vi "split_averaging_filter_cdb.vi"(4 "Reset":bool, 8 "Parameters":T1={"Order"=0, "Time constant"=0.0, "Detrend mode"=enum."Robust linear", "TD amplitude limit"=inf, "FFT filter"=TRUE, "Notch channels"=[], "LF cutoff"=0, "FD amplitude limit"=0.0}, 9 "Noise":bool, 11 "Error":cdb[](array[numeric])) -> (1 "Model":cdb[](array[numeric]) format="%#_3p", 3 "Prediction":cdb[](array[numeric]) format="%#_4p")   [LabVIEW 2014]
uses:
  averaging_filter_params.ctl
  detrend_mode.ctl
panel:
  # "Prediction for next data block, the same size as our input this time."
  # "The filter tracking error (what we are to try to cancel)."
  # "The time domain model, with length \"Order\".   This is synchronous with the repeat period."
  # "If true, our adaptation should be suppressed on this \"Signal\" block."
  # "This is derived from split_averaging_filter_nu.vi, but has been modified to work with complex input/output data, with inputs that have DC component, and some unused features have also been deleted."
  # "Reset clears state to zeroes.  Filter must then settle to the steady-state output (multiple time constants)."
  # "Model of a repeating signal with known repeat period (order).  Input may be any length; prediction is the same size as input, while the model is of the specified order.  This is like the averaging function on an oscilloscope.  As long as the time constant is much longer than the filter order, only signals that are synchronous with the order pass through into the model."
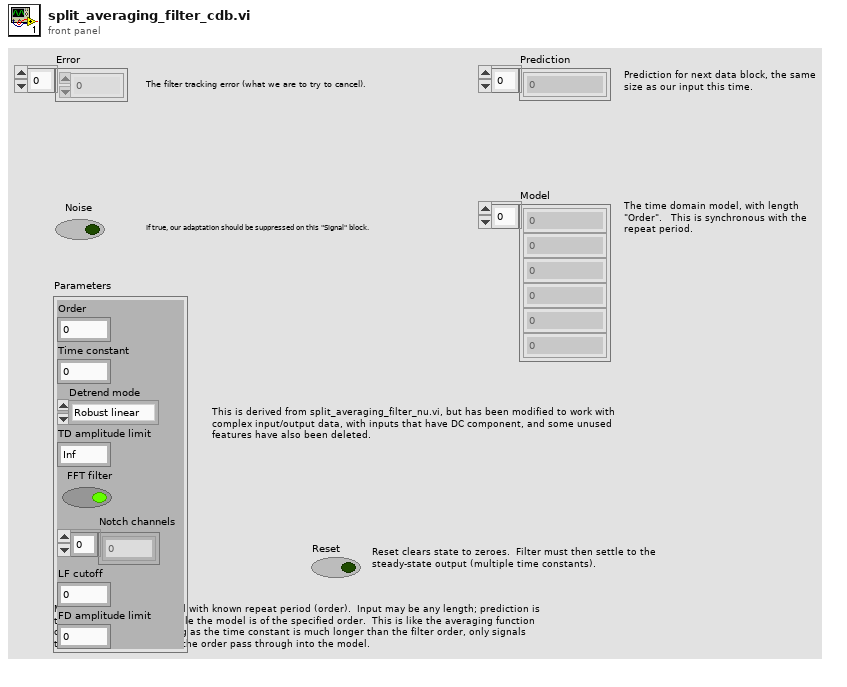
[diagram p1: front panel]
types:
  T1 = typedef "averaging_filter_params.ctl" = cluster{"Order":i32, "Time constant":dbl, "Detrend mode":T2, "TD amplitude limit":dbl, "FFT filter":bool, "Notch channels":i32[], "LF cutoff":i32, "FD amplitude limit":dbl}
  T2 = typedef "detrend_mode.ctl" = enum16{"Zero mean", "Linear", "Robust linear"}
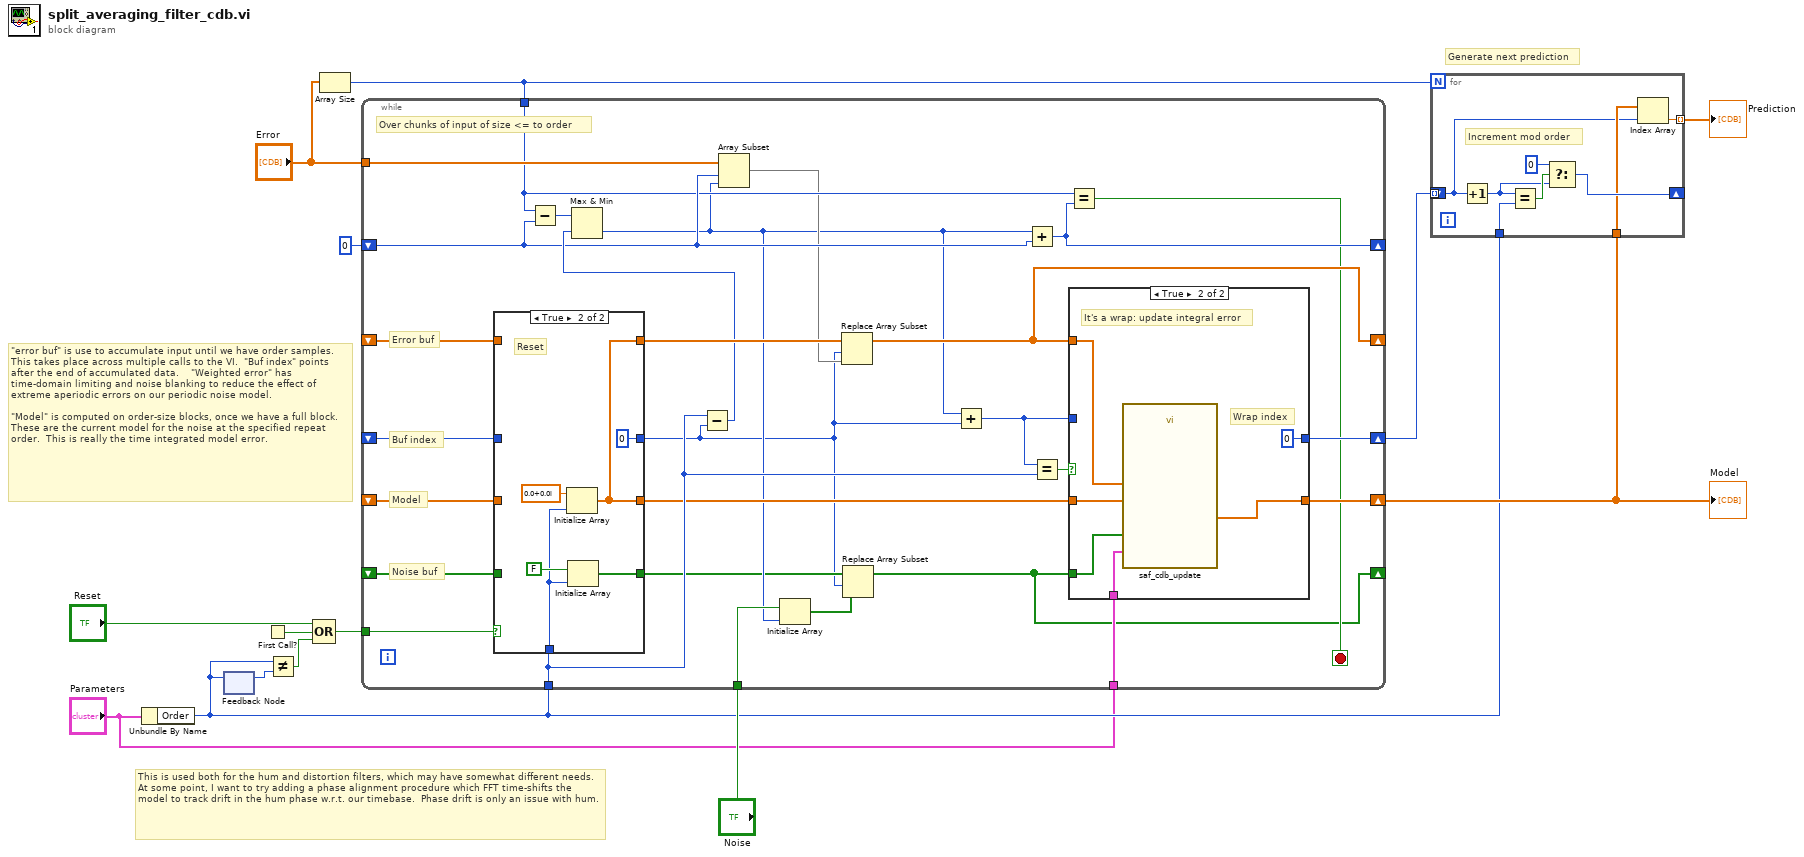
[diagram p0: block diagram]
diagram:
  # "Generate next prediction"
  # "\"error buf\" is use to accumulate input until we have order samples.  This takes place across multiple calls to the VI.  \"Buf index\" points after the end of accumulated data.    \"Weighted error\" has time-domain limiting and noise blanking to reduce the effect of extreme aperiodic errors on our periodic noise model. \n\n\"Model\" is computed on order-size blocks, once we have a full block.  These are the current model for the noise at the specified repeat order.  This is really the time integrated model error."
  # "This is used both for the hum and distortion filters, which may have somewhat different needs.  At some point, I want to try adding a phase alignment procedure which FFT time-shifts the model to track drift in the hum phase w.r.t. our timebase.  Phase drift is only an issue with hum."
  n1 = Unbundle By Name("Parameters") -> ("Order"=w10:i32)
  n2 = feedback-in #1(w10) -> ()
  n3 = feedback #1() -> (w11:i32)  [unwired: 1 in]
  n4 = First Call?() -> (First Call?: T/F=w14:bool)
  n5 = Not Equal?(x=w10, y=w11) -> (x != y?=w9:bool)
  n6 = Compound Arithmetic op=OR("Reset", w14, w9) -> (w8:bool)
  n7 = Array Size(array="Error") -> (size(s)=w5:i32)
  n8 = while {
    shift-right: [w42] -> w7
    shift-left: _ -> [w36]
    tunnel: w10 -> [w25]
    shift-right: [w40] -> w13
    shift-left: _ -> [w39]
    shift-right: [w31] -> _
    shift-left: _ -> [w37]
    tunnel: "Parameters" -> [w41]
    tunnel: "Noise" -> [w20]
    tunnel: w8 -> [w38]
    tunnel: "Error" -> [w34]
    shift-right: [w27] -> _
    shift-left: 0 ("Order") -> [w29]
    tunnel: w5 -> [w28]
    shift-right: [w15] -> _
    shift-left: _ -> [w22]
    stop <- w26 stop-if-true
    # "Noise buf"
    # "Over chunks of input of size <= to order"
    # "Buf index"
    # "Error buf"
    # "Model"
    n9 = case shown="True" w38 {
      tunnel: w25 -> [_ w48]
      tunnel: [w46 w50] -> w24
      tunnel: w39 -> [w46 _]
      tunnel: [w44 0 ("Order")] -> w16
      tunnel: [w45 w50] -> w33
      tunnel: w37 -> [w45 _]
      tunnel: w36 -> [w44 _]
      tunnel: w22 -> [w43 _]
      tunnel: [w43 w47] -> w17
      frame False {
        # "Not reset"
      }
      frame True {
        # "Reset"
        n10 = Initialize Array(cdb 0.0+0.0i ("Decay"), w48) -> (w50:cdb[])
        n11 = Initialize Array(FALSE, w48) -> (w47:bool[])
      }
    }
    n12 = Subtract(x=w28, y=w29) -> (x-y=w35:i32)
    n13 = Subtract(x=w25, y=w16) -> (x-y=w32:i32)
    n14 = Max & Min(x=w35, y=w32) -> (min(x,y)=w19:i32)  [unwired: 1 out]
    n15 = Array Subset(array=w34, index=w29, length=w19) -> (w21:cdb[])
    n16 = Initialize Array(w20, w19) -> (w18:bool[])
    n17 = Replace Array Subset(array=w33, new element=w21, index=w16) -> (w31:cdb[])
    n18 = Replace Array Subset(array=w17, new element=w18, index=w16) -> (w15:bool[])
    n19 = Add(x=w19, y=w16) -> (x+y=w30:i32)
    n20 = Add(x=w19, y=w29) -> (x+y=w27:i32)
    n21 = Equal?(x=w30, y=w25) -> (x = y?=w23:bool)
    n22 = Equal?(x=w28, y=w27) -> (x = y?=w26:bool)
    n23 = case shown="True" w23 {
      tunnel: [w53 0] -> w42
      tunnel: w30 -> [w53 _]
      tunnel: w31 -> [_ w56]
      tunnel: w41 -> [_ w57]
      tunnel: [w54 w59] -> w40
      tunnel: w24 -> [w54 w58]
      tunnel: w15 -> [_ w55]
      frame False {
        # "Not a wrap"
      }
      frame True {
        # "Wrap index"
        # "It's a wrap: update integral error"
        n24 = call "saf_cdb_update.vi"("Noise"=w55, "Parameters"=w57, "Model"=w58, "Buffer"=w56) -> ("New model"=w59:cdb[])  [unwired: 7 in]
      }
    }
  }
  "Model" <- w13
  n25 = for {
    N: w5 -> [_]
    shift-right: [w64] -> _
    shift-left: w7 -> [w61]
    tunnel: w10 -> [w67]
    tunnel: [w63] -> w4 mode=indexing
    tunnel: w13 -> [w62]
    tunnel: [w61] -> _ mode=indexing
    # "Increment mod order"
    n26 = Increment(x=w61) -> (x+1=w66:i32)
    n27 = Equal?(x=w66, y=w67) -> (x = y?=w68:bool)
    n28 = Select(t=0, s=w68, f=w66) -> (s? t:f=w64:i32)
    n29 = Index Array(array=w62, index=w61) -> (element=w63:cdb)
  }
  "Prediction" <- w4
